vi "Get Multipart Upload ID.vi"(8 "error in (no error)":errorcluster, 11 "Multipart Upload RefNum in":T1) -> (0 "error out":errorcluster, 2 "Upload ID":string, 3 "Multipart Upload RefNum out":T1)   [LabVIEW 2015, in "LV Interface for Amazon S3.lvlib"]
doc: "Use this VI to get the unique <B>Upload ID associated with a multipart upload</B> already started. You can <B>use the Upload ID to list the parts</B> already uploaded (see List Parts.vi)."
uses:
  LV Interface for Amazon S3.lvlib
  Typedefs/AMZ_S3_Multipart Upload RefNum.ctl
  Typedefs/AMZ_S3_Multipart Upload RefNum Enum.ctl
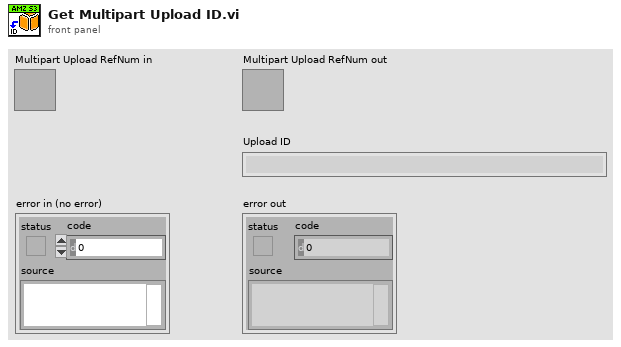
[diagram p1: front panel]
types:
  T1 = typedef "LV Interface for Amazon S3.lvlib/AMZ_S3_Multipart Upload RefNum.ctl" = refnum<k1>
  T2 = typedef "LV Interface for Amazon S3.lvlib/AMZ_S3_Multipart Upload Data.ctl" = cluster{"Object":string, "Bucket":string, "UploadID":string, "Parts":T3[]}
  T3 = typedef "LV Interface for Amazon S3.lvlib/AMZ_S3_Multipart Upload Part Data.ctl" = cluster{"PartNumber":u16, "Lat modified":timestamp, "ETag":string, "Size":u64}
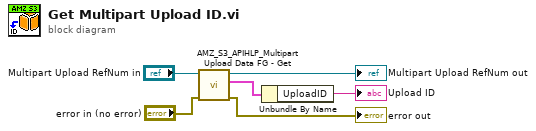
[diagram p0: block diagram]
diagram:
  n1 = call "AMZ_S3_APIHLP_Multipart Upload Data FG - Get.vi"("error in (no error)"="error in (no error)", "Multipart Upload RefNum in"="Multipart Upload RefNum in") -> ("error out"=→"error out":errorcluster, "Multipart Upload Data"=w2:T2, "Multipart Upload RefNum out"=→"Multipart Upload RefNum out":T1)  [unwired: 7 in]
  n2 = Unbundle By Name(w2) -> ("UploadID"=→"Upload ID":string)
